vi "Read Instrument Setting.vi"(8 "error in (no error)":errorcluster, 11 "Instrument configuration in":refnum<class "Instrument configuration.lvclass">) -> (0 "error out":errorcluster, 2 "Instrument Setting":T1={"Type"="None", "Address"="localhost", "SW Alias"="Type = Class \n", "Description"="1.0.0.0", "Enabled"=TRUE}, 3 "Instrument configuration out":refnum<class "Instrument configuration.lvclass">)   [LabVIEW 2025, in "Abstract Engine.lvlib" / "Instrument configuration.lvclass"]
uses:
  Instrument configuration.lvclass
  Instrument configuration.lvclass/Instrument configuration.ctl
  Default Instrument.ctl
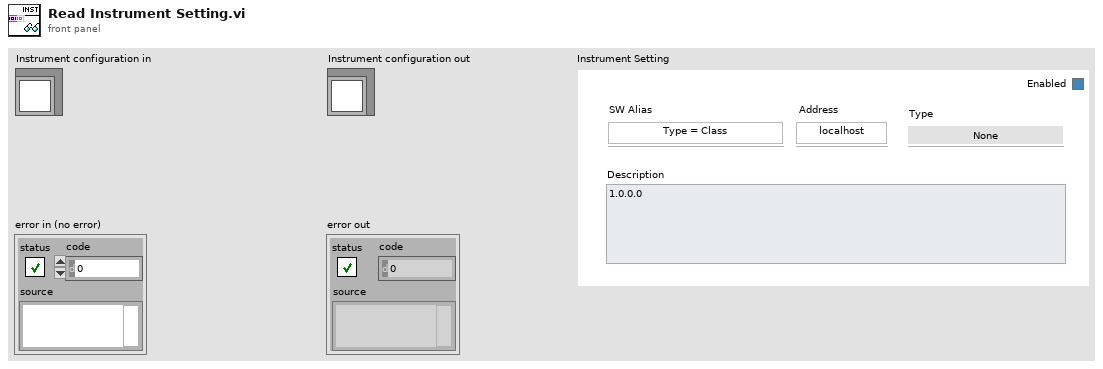
[diagram p1: front panel]
types:
  T1 = typedef "Abstract Engine.lvlib/Instrument configuration.lvclass/Default Instrument.ctl" = cluster{"Type":string, "Address":string, "SW Alias":string, "Description":string, "Enabled":bool}
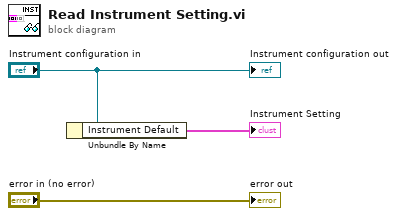
[diagram p0: block diagram]
diagram:
  n1 = Unbundle By Name("Instrument configuration in") -> ("Instrument Default"=→"Instrument Setting":T1)
  "error out" <- "error in (no error)"
  "Instrument configuration out" <- "Instrument configuration in"
